vi "CLC_JIO_subBFIC_channel.vi"(8 "error in":errorcluster, 11 "JIO--channel":T1={"Disable"=1, "T/R Mode"=0, "Ch_Index"=1, "IC_Index"=1, "Chain"=1, "Phase"=0, "ELE Gain"=0, "Com Gain"=0, "H/V Polarity"=0} {"Disable" max=1; "T/R Mode" max=1; "Ch_Index" min=1 max=4; "IC_Index" min=1 max=4; "Chain" min=1 max=2; "Phase" max=63; "ELE Gain" max=15; "Com Gain" max=15; "H/V Polarity" max=1}) -> (0 "error out":errorcluster, 3 "standard output":string)   [LabVIEW 2023, in "CLC_JIO_FTDI.lvlib"]
uses:
  CLC_JIO_FTDI.lvlib
panel:
  out "resulting string":string
  out "appended path":path
  out "standard error":string
  out "Check driver floder?":bool
  # "1-2"
  # "1-4"
  # "1-4"
  # "0:Tx\n1:Rx"
  # "0:H\n1:V"
  # "0:On\n1:OFF"
  # "0-15"
  # "0-15"
  # "0-15"
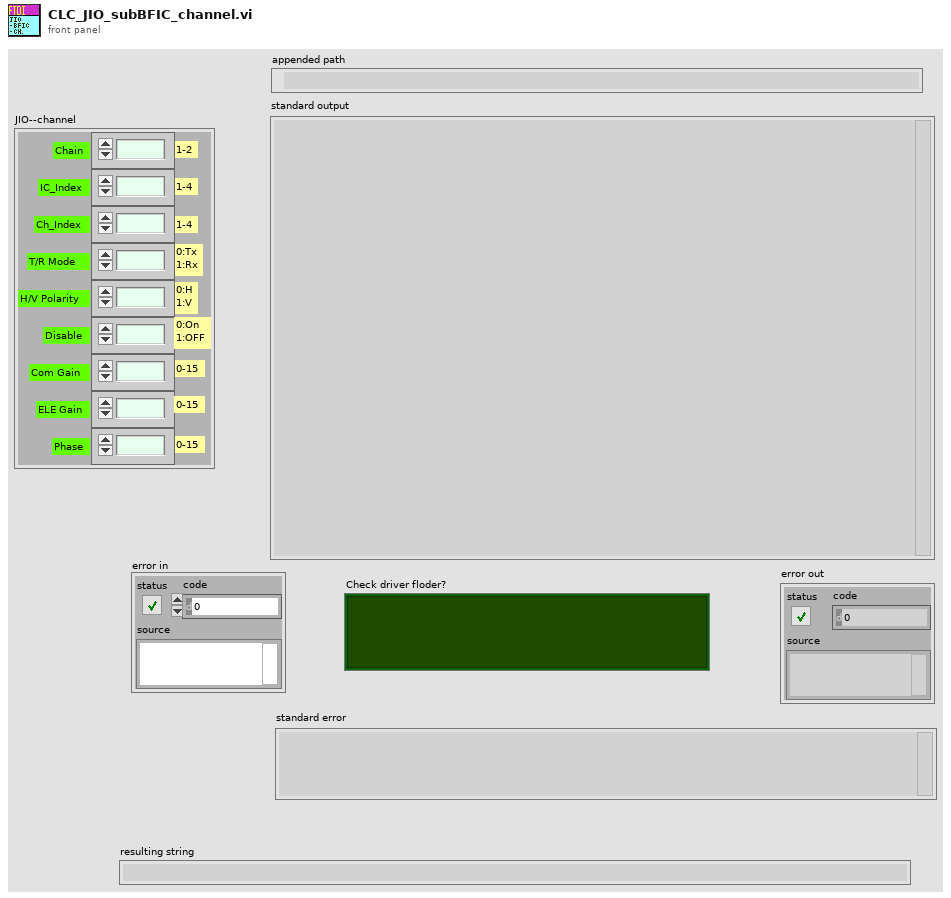
[diagram p1: front panel]
types:
  T1 = cluster{"Disable":u16, "T/R Mode":u16, "Ch_Index":u16, "IC_Index":u16, "Chain":u16, "Phase":u16, "ELE Gain":u16, "Com Gain":u16, "H/V Polarity":u16}
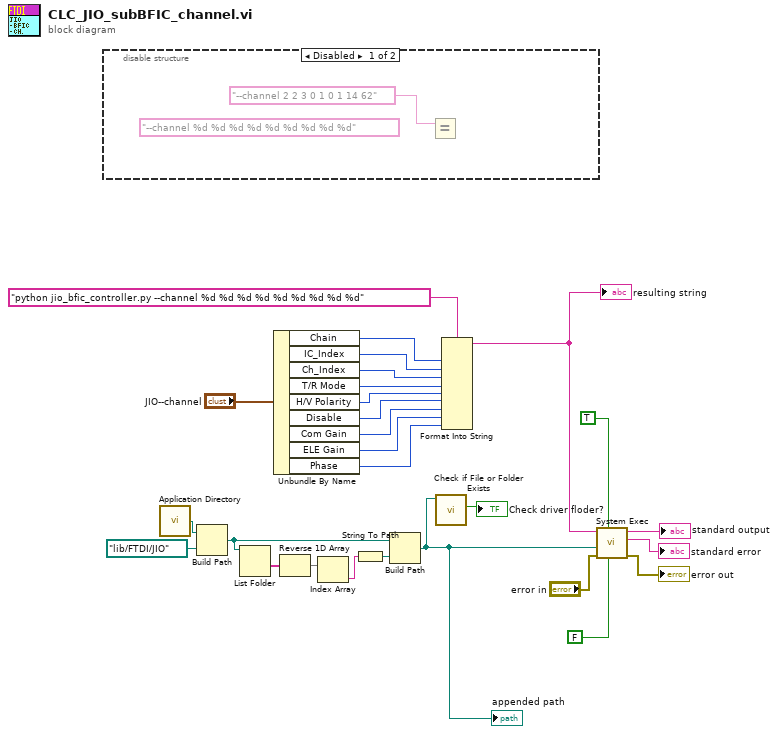
[diagram p0: block diagram]
diagram:
  n1 = disable-structure shown="Disabled" {
    frame Disabled {
      (unwired) "--channel %d %d %d %d %d %d %d %d %d" ("command line")
      n2 = Equal?(x="--channel 2 2 3 0 1 0 1 14 62") -> ()  [unwired: 1 in, 1 out]
    }
    frame Enabled {
    }
  }
  n3 = call <vilib>:"Application Directory.vi"() -> ("Application Directory"=w21:path)
  n4 = Build Path(base path=w21, name or relative path=path "lib/FTDI/JIO") -> (appended path=w20:path)
  n5 = List Folder(path=w20) -> (folder names=w26:string[])  [unwired: 3 in, 3 out]
  n6 = Unbundle By Name("JIO--channel") -> ("Chain"=w11:u16, "IC_Index"=w10:u16, "Ch_Index"=w9:u16, "T/R Mode"=w8:u16, "H/V Polarity"=w7:u16, "Disable"=w6:u16, "Com Gain"=w5:u16, "ELE Gain"=w4:u16, "Phase"=w3:u16)
  n7 = Reverse 1D Array(array=w26) -> (reversed array=w25:string[])
  n8 = Index Array(array=w25) -> (element=w24:string)  [unwired: 1 in]
  n9 = String To Path(string=w24) -> (path=w23:path)
  n10 = Build Path(base path=w20, name or relative path=w23) -> (appended path=w18:path)
  "appended path" <- w18
  n11 = call <vilib>:"Check if File or Folder Exists.vi"("path"=w18) -> ("file or folder exists?"=→"Check driver floder?":bool)  [unwired: 8 in, 2 out]
  n12 = Format Into String(format string="python jio_bfic_controller.py --channel %d %d %d %d %d %d %d %d %d" ("command line"), w11, w10, w9, w8, w7, w6, w5, w4, w3) -> (resulting string=w2:string)  [unwired: 2 in, 1 out]
  "resulting string" <- w2
  n13 = call <vilib>:"System Exec.vi"("run minimized? (F)"=FALSE, "wait until completion? (T)"=TRUE, "error in (no error)"="error in", "working directory"=w18, "command line"=w2) -> ("error out"=→"error out":errorcluster, "standard error"=→"standard error":string, "standard output"=→"standard output":string)  [unwired: 3 in, 1 out]
